vi "Do.vi"(8 "error in (no error)":errorcluster, 10 "Actor in":refnum<class "Actor.lvclass">, 11 "Integration Start Stop Msg":refnum<class "Integration Start Stop Msg.lvclass">) -> (0 "error out":errorcluster, 2 "Actor out":refnum<class "Actor.lvclass">)   [LabVIEW 2012, in "Universal Power Meter.lvlib" / "WT1600.lvlib" / "Integration Start Stop Msg.lvclass"]
doc: "This VI delivers the message to the actor by calling the appropriate method(s) on the actor."
uses:
  Integration Start Stop Msg.lvclass
  <vilib>/ActorFramework/Actor/Actor.lvclass
  WT1600/WT1600.lvclass
  Integration Start Stop Msg.lvclass/Integration Start Stop Msg.ctl
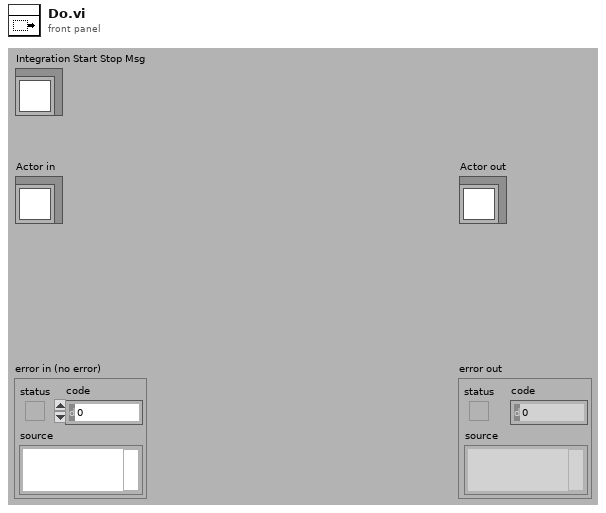
[diagram p1: front panel]
types:
  T1 = enum16{"All", "Element 1", "Element 2", "Element 3", "Element 4", "Element 5", "Element 6"}
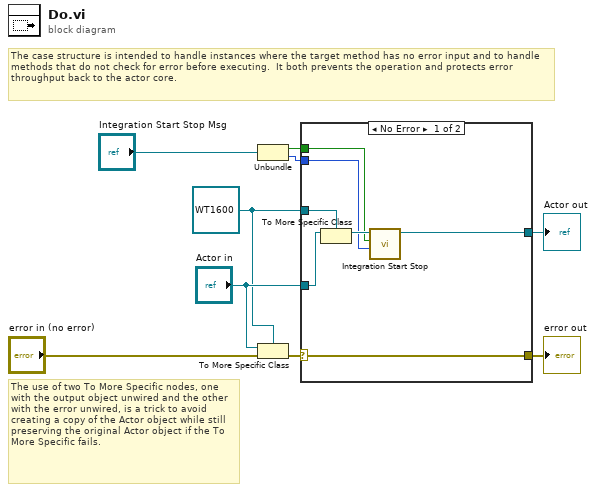
[diagram p0: block diagram]
diagram:
  w3 = refnum<class "WT1600.lvclass"> refnum ("Actor in")
  # "The use of two To More Specific nodes, one with the output object unwired and the other with the error unwired, is a trick to avoid creating a copy of the Actor object while still preserving the original Actor object if the To More Specific fails."
  # "The case structure is intended to handle instances where the target method has no error input and to handle methods that do not check for error before executing.  It both prevents the operation and protects error throughput back to the actor core."
  n1 = Unbundle("Integration Start Stop Msg") -> (w2:bool, w1:T1)
  n2 = To More Specific Class(target class=w3, reference="Actor in", error in="error in (no error)") -> (error out=w7:errorcluster)  [unwired: 1 out]
  n3 = case shown="No Error" w7 {
    selector: w7 -> [w15 w18]
    tunnel: [w15 w18] -> w6
    tunnel: [w16 w17] -> w5
    tunnel: "Actor in" -> [w14 w17]
    tunnel: w3 -> [w13 _]
    tunnel: w2 -> [w11 _]
    tunnel: w1 -> [w10 _]
    frame No Error {
      n4 = To More Specific Class(target class=w13, reference=w14) -> (specific class reference=w12:refnum<class "WT1600.lvclass">)  [unwired: 1 in, 1 out]
      n5 = call "Integration Start Stop.vi"("Element (All: 0)"=w10, "Start/Stop (F: Stop)"=w11, "WT1600.lvlib:WT1600.lvclass"=w12) -> ("WT1600 out"=w16:refnum<class "WT1600.lvclass">)  [unwired: 8 in]
    }
    frame Error {
      # "If type check fails, pass the original object out again."
    }
  }
  "error out" <- w6
  "Actor out" <- w5
